vi "ma_HasarrIIRSpecsChanged.vi"(4 "optional IIR filter specifications":T1(array[cluster]) {"PB Gain" format="%0.2f"; "SB Gain" format="%0.2f"; "Lower SB" format="%0.2p"; "Upper SB" format="%0.2f"; "Lower PB" format="%0.2p"; "Upper PB" format="%0.2f"}, 6 "IIR filter specs":T2(array[cluster]) {"PB Ripple" format="%0.2f"; "Lower Fc" format="%0.2p"; "SB Attenuation" format="%0.2f"; "Upper Fc" format="%0.2p"}, 8 "error in (no error)":errorcluster, 10 "redesign filter":bool[](array[boolean])) -> (0 "error out":errorcluster, 3 "valsDifferent?":bool[](array[boolean]))   [LabVIEW 2020, in "NI_MAPro.lvlib"]
uses:
  NI_MAPro.lvlib
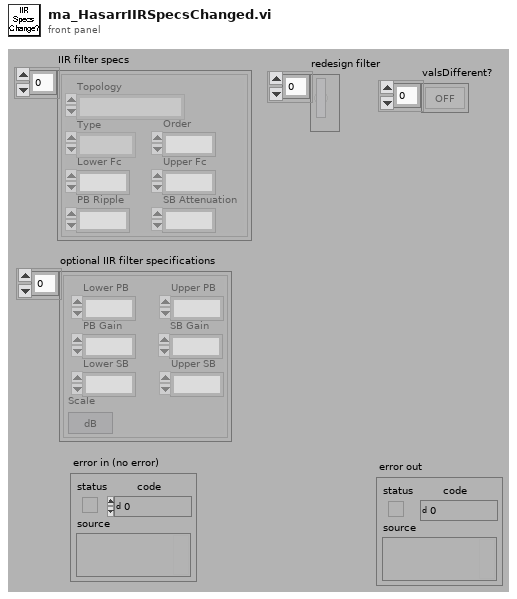
[diagram p1: front panel]
types:
  T1 = cluster{"Lower PB":dbl, "Upper PB":dbl, "Lower SB":dbl, "Upper SB":dbl, "PB Gain":dbl, "SB Gain":dbl, "Scale":bool}[]
  T2 = cluster{"Topology":enum16{"Off", "Butterworth", "Chebyshev", "Inverse Chebyshev", "Elliptic", "Bessel"}, "Type":enum16{"Lowpass", "Highpass", "Bandpass", "Bandstop"}, "Order":i32, "Lower Fc":dbl, "Upper Fc":dbl, "PB Ripple":dbl, "SB Attenuation":dbl}[]
  T3 = cluster{"Topology":enum16{"Off", "Butterworth", "Chebyshev", "Inverse Chebyshev", "Elliptic", "Bessel"}, "Type":enum16{"Lowpass", "Highpass", "Bandpass", "Bandstop"}, "Order":i32, "Lower Fc":dbl, "Upper Fc":dbl, "PB Ripple":dbl, "SB Attenuation":dbl}
  T4 = cluster{"Lower PB":dbl, "Upper PB":dbl, "Lower SB":dbl, "Upper SB":dbl, "PB Gain":dbl, "SB Gain":dbl, "Scale":bool}
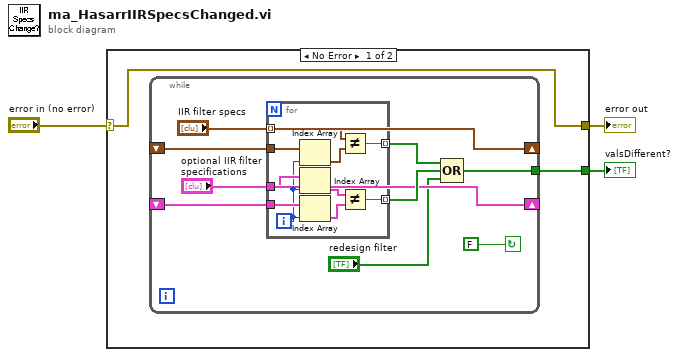
[diagram p0: block diagram]
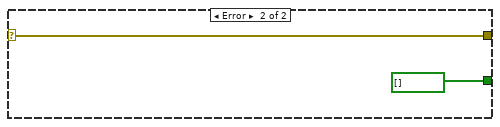
[diagram p2: hidden frame]
diagram:
  n1 = case shown="No Error" "error in (no error)" {
    selector: "error in (no error)" -> [w4 w26]
    tunnel: [w5 bool[] [] ("Array Constant")] -> w1
    tunnel: [w4 w26] -> w2
    frame No Error {
      n2 = while {
        shift-left: _ -> [w13]
        shift-right: ["optional IIR filter specifications"] -> _
        tunnel: [w9] -> w5
        shift-left: _ -> [w12]
        shift-right: ["IIR filter specs"] -> _
        stop <- FALSE continue-if-true
        n3 = for {
          tunnel: w13 -> [w21]
          tunnel: w12 -> [w18]
          tunnel: [w24] -> w11 mode=indexing
          tunnel: [w23] -> w10 mode=indexing
          tunnel: "IIR filter specs" -> [w22] mode=indexing
          tunnel: "optional IIR filter specifications" -> [w16]
          i -> [w15]
          n4 = Index Array(array=w18, index=w15) -> (element=w19:T3)
          n5 = Index Array(array=w16, index=w15) -> (element=w17:T4)
          n6 = Index Array(array=w21, index=w15) -> (element=w20:T4)
          n7 = Not Equal?(x=w22, y=w19) -> (x != y?=w24:bool)
          n8 = Not Equal?(x=w17, y=w20) -> (x != y?=w23:bool)
        }
        n9 = Compound Arithmetic op=OR(w11, w10, "redesign filter") -> (w9:bool[])
      }
    }
    frame Error {
    }
  }
  "error out" <- w2
  "valsDifferent?" <- w1
